vi "Configure Mask Scaling.vi"(8 "error in (no error)":errorcluster, 9 "Horizontal Scaling":T2 {"Delta X (118E-9 s)" format="%^#_6g"}, 10 "Vertical Scaling":T1, 11 "VISA resource name":refnum<visa-resource-name>) -> (0 "error out":errorcluster, 3 "VISA resource name out":refnum<visa-resource-name>)   [LabVIEW 2009, in "Agilent 8000 Series.lvlib"]
doc: "Configures the mask scaling parameters.\n\n<b>Note: </b>\n\nMask testing must be enabled for this VI to operate or a \"Settings Conflict\" error might be thrown. This can be done through the \"Configure Mask Test\" VI."
uses:
  Agilent 8000 Series.lvlib
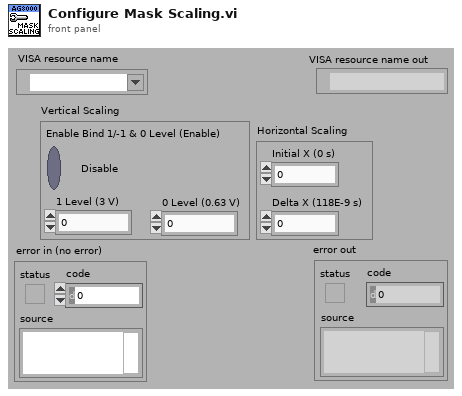
[diagram p1: front panel]
types:
  T1 = cluster{"Enable Bind 1/-1 & 0 Level (Enable)":bool, "1 Level (3 V)":dbl, "0 Level (0.63 V)":dbl}
  T2 = cluster{"Initial X (0 s)":dbl, "Delta X (118E-9 s)":dbl}
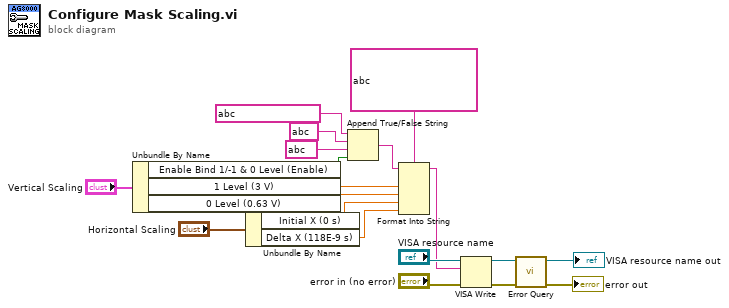
[diagram p0: block diagram]
diagram:
  n1 = Unbundle By Name("Vertical Scaling") -> ("Enable Bind 1/-1 & 0 Level (Enable)"=w5:bool, "1 Level (3 V)"=w4:dbl, "0 Level (0.63 V)"=w3:dbl)
  n2 = Unbundle By Name("Horizontal Scaling") -> ("Initial X (0 s)"=w2:dbl, "Delta X (118E-9 s)"=w1:dbl)
  n3 = Append True/False String(1:w5, 2:string ? ("false string"), 3:string ? ("true string"), 4:string ? ("string (\"\")")) -> (0:w10:string)
  n4 = Format Into String(format string=string ?, initial string=w10, w4, w3, w2, w1) -> (resulting string=w9:string)  [unwired: 1 in, 1 out]
  n5 = VISA Write(VISA resource name="VISA resource name", write buffer=w9, error in (no error)="error in (no error)") -> (VISA resource name out=w17:refnum<visa-resource-name>, error out=w16:errorcluster)  [unwired: 1 out]
  n6 = call "Error Query.vi"("error in (no error)"=w16, "VISA resource name"=w17) -> ("error out"=→"error out":errorcluster, "VISA resource name out"=→"VISA resource name out":refnum<visa-resource-name>)  [unwired: 6 in, 2 out]
